vi "test ellipse svd.vi"() -> ()   [LabVIEW 2017]
uses:
  <vilib>/gmath/statdist.llb/Normal Random.vi
  <vilib>/gmath/NI_Gmath.lvlib
panel:
  out "XY Graph":cluster{"X":dbl[], "Y":dbl[]}[](graph)
  out "ellipse parameters 2":T1
  in  "sigma noise":dbl=1.0
  in  "ellipse parameters":T1
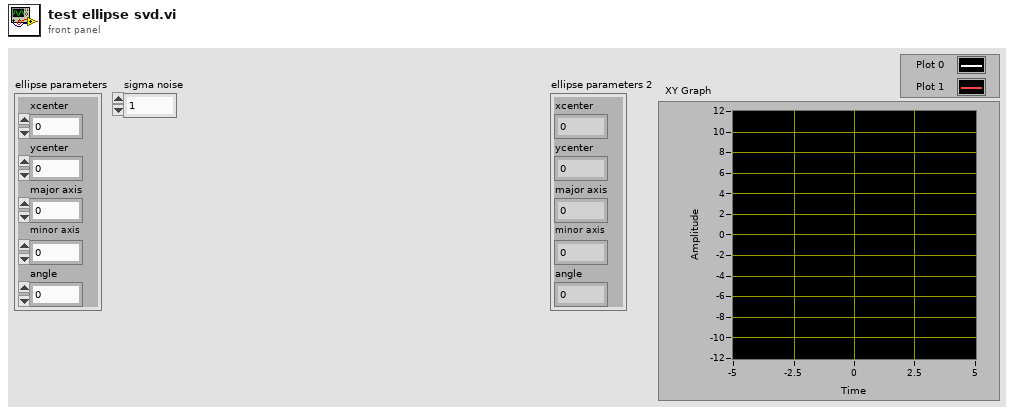
[diagram p1: front panel]
types:
  T1 = cluster{"xcenter":dbl, "ycenter":dbl, "major axis":dbl, "minor axis":dbl, "angle":dbl}
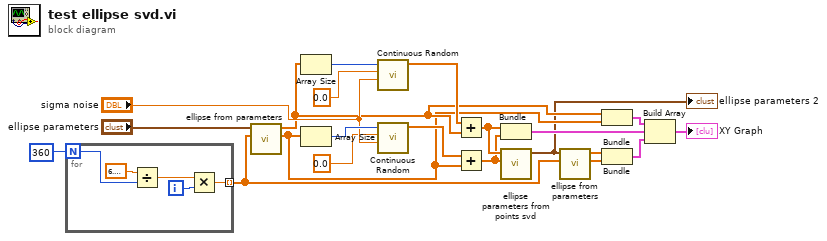
[diagram p0: block diagram]
diagram:
  n1 = for {
    N: 360 -> [w24]
    tunnel: [w22] -> w4 mode=indexing
    i -> [w26]
    n2 = Divide(x=6.283185307179586, y=w24) -> (x/y=w23:dbl)
    n3 = Multiply(x=w23, y=w26) -> (x*y=w22:dbl)
  }
  n4 = call "ellipse from parameters.vi"("phi"=w4, "ellipse parameters"="ellipse parameters") -> ("Y"=w11:dbl[], "X"=w12:dbl[])  [unwired: 8 in]
  n5 = Array Size(array=w12) -> (size(s)=w18:i32)
  n6 = Array Size(array=w11) -> (size(s)=w17:i32)
  n7 = call-poly <vilib>:"Continuous Random.vi"("std"="sigma noise", "mean"=0.0, "samples"=w18) -> ("normal random data"=w14:dbl[])  [unwired: 7 in, 1 out]
  n8 = call-poly <vilib>:"Continuous Random.vi"("std"="sigma noise", "mean"=0.0, "samples"=w17) -> ("normal random data"=w13:dbl[])  [unwired: 7 in, 1 out]
  n9 = Add(x=w14, y=w12) -> (x+y=w9:dbl[])
  n10 = Add(x=w13, y=w11) -> (x+y=w8:dbl[])
  n11 = Bundle(w9, w8) -> (w6:cluster{dbl[], dbl[]})  [unwired: 1 in]
  n12 = call "ellipse parameters from points svd.vi"("y"=w8, "X"=w9) -> ("ellipse parameters"=w5:T1)  [unwired: 9 in]
  "ellipse parameters 2" <- w5
  n13 = call "ellipse from parameters.vi"("phi"=w4, "ellipse parameters"=w5) -> ("Y"=w2:dbl[], "X"=w3:dbl[])  [unwired: 8 in]
  n14 = Bundle("X"=w12, "Y"=w11) -> (w10:cluster{"X":dbl[], "Y":dbl[]})  [unwired: 1 in]
  n15 = Bundle("X"=w3, "Y"=w2) -> (w1:cluster{"X":dbl[], "Y":dbl[]})  [unwired: 1 in]
  n16 = Build Array(w10, w6, w1) -> (→"XY Graph":cluster{"X":dbl[], "Y":dbl[]}[])
